vi "Dax_RadValsBP1.vi"(11 "Daxsonics":refnum<visa-resource-name>) -> (0 "Dax Values":cluster{"Freq":i32, "Amp":i32, "Gain":i32}, 1 "Freq (MHz)":u16=1, 2 "Amp (V)":u16, 3 "Gain (dB)":u16)   [LabVIEW 2022 SP3]
uses:
  ScanningControl/Pulsers/PulserGlobals.vi
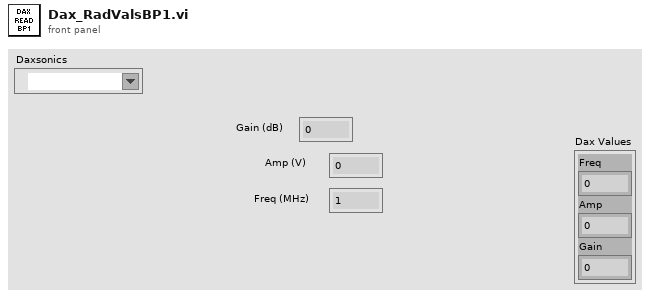
[diagram p1: front panel]
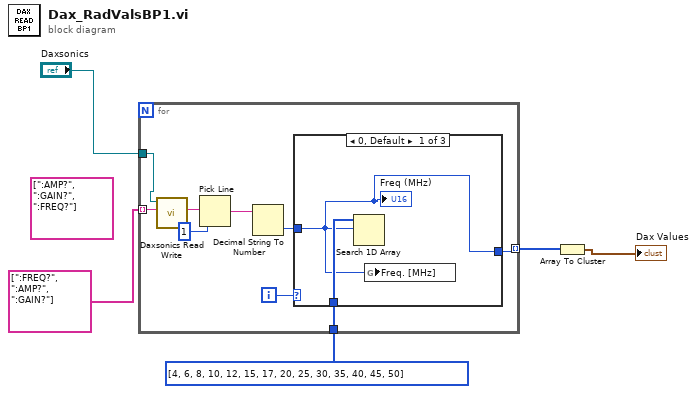
[diagram p0: block diagram]
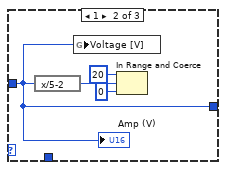
[diagram p2: hidden frame]
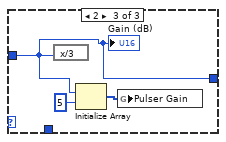
[diagram p3: hidden frame]
diagram:
  (unwired) string[] [":AMP?", ":GAIN?", ":FREQ?"]
  n1 = for {
    tunnel: string[] [":FREQ?", ":AMP?", ":GAIN?"] -> [w11] mode=indexing
    tunnel: i32[] [4, 6, 8, 10, 12, 15, 17, 20, 25, 30, 35, 40, 45, 50] -> [w12]
    tunnel: "Daxsonics" -> [w7]
    tunnel: [w6] -> w3 mode=indexing
    i -> [w14]
    n2 = call "Daxsonics Read Write.vi"("write buffer"=w11, "VISA resource name"=w7) -> ("read buffer"=w10:string)  [unwired: 7 in, 2 out]
    n3 = Pick Line(multi-line string=w10, line index=1) -> (output string=w9:string)  [unwired: 1 in]
    n4 = Decimal String To Number(string=w9) -> (number=w13:i32)  [unwired: 2 in, 1 out]
    n5 = case shown="0, Default" w14 {
      tunnel: w13 -> [w15 w17 w22]
      tunnel: w12 -> [w16 _ _]
      tunnel: [w15 w17 w22] -> w6
      frame 0, Default {
        n6 = Search 1D Array(1D array=w16, element=w15) -> ()  [unwired: 1 in, 1 out]
        n7 = global write "PulserGlobals.vi" "Freq. [MHz]"(w15) -> ()
        "Freq (MHz)" <- w15
      }
      frame 1 {
        n8 = expression code="x/5-2"(w17) -> (w20:i32)
        n9 = global write "PulserGlobals.vi" "Voltage [V]"(w17) -> ()
        n10 = In Range and Coerce(upper limit=20, x=w20, lower limit=0) -> ()  [unwired: 2 out]
        "Amp (V)" <- w17
      }
      frame 2 {
        n11 = expression code="x/3"(w22) -> ()  [unwired: 1 out]
        n12 = Initialize Array(w22, 5 ("dimension size")) -> (w21:i32[])
        n13 = global write "PulserGlobals.vi" "Pulser Gain"(w21) -> ()
        "Gain (dB)" <- w22
      }
    }
  }
  n14 = Array To Cluster(array=w3) -> (cluster=→"Dax Values":cluster{"[0]":i32, "[1]":i32, "[2]":i32})
